vi "Home_String_to_Enumerated_Type.vi"(1 "String":string) -> (0 "Home":T1)   [LabVIEW 2022 SP3]
uses:
  Controls/Home.ctl
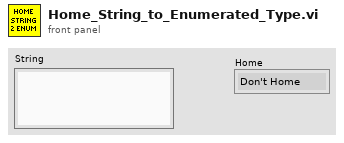
[diagram p1: front panel]
types:
  T1 = typedef "Home.ctl" = enum16{"Don't Home", "Home  +X", "Home  -X", "Home  +Y", "Home  -Y", "Home  +Z", "Home  -Z"}
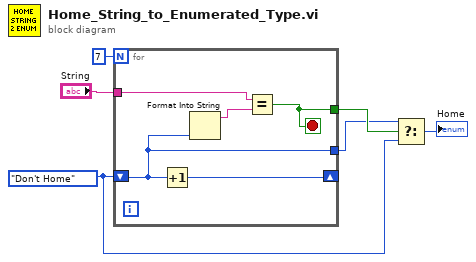
[diagram p0: block diagram]
diagram:
  w2 = Home."Don't Home" ("Home")
  n1 = for {
    N: 7 -> [_]
    shift-right: [w11] -> _
    shift-left: w2 -> [w8]
    tunnel: "String" -> [w9]
    tunnel: [w8] -> w3
    tunnel: [w7] -> w4
    stop <- w7 stop-if-true
    n2 = Increment(x=w8) -> (x+1=w11:T1)
    n3 = Format Into String(w8) -> (resulting string=w10:string)  [unwired: 3 in, 1 out]
    n4 = Equal?(x=w9, y=w10) -> (x = y?=w7:bool)
  }
  n5 = Select(t=w3, s=w4, f=w2) -> (s? t:f=→"Home":T1)
